vi "导出曲线数组.vi"(9 "file path (dialog if empty)":path caption="文件路径 （空时为对话框）", 10 "数组 2":dbl[](array[numeric]), 11 "数组":dbl[](array[numeric])) -> ()   [LabVIEW 2013]
uses:
  <vilib>/Utility/file.llb/Write To Spreadsheet File (DBL).vi
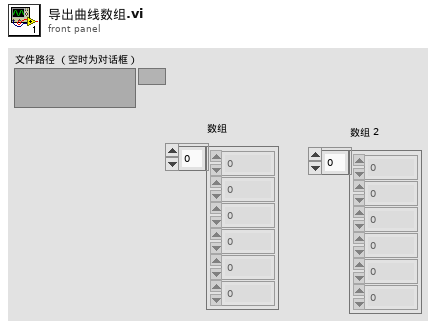
[diagram p1: front panel]
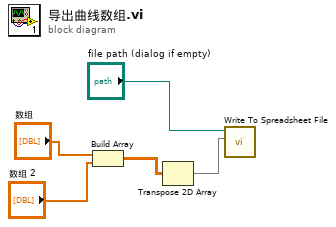
[diagram p0: block diagram]
diagram:
  n1 = Build Array("数组", "数组 2") -> (w3:dbl[][])
  n2 = Transpose 2D Array(2D array=w3) -> (transposed array=w2:dbl[][])
  n3 = call-poly <vilib>:"Write To Spreadsheet File.vi"("2D data"=w2, "file path (dialog if empty)"="file path (dialog if empty)") -> ()  [unwired: 6 in, 1 out]
